vi "CheckUserPass.vi"(6 "password":string, 7 "user":string, 8 "error in":errorcluster, 9 "PasswordRecieved":string, 10 "UserRecieved":string, 11 "connection ID in":refnum<k5>) -> (0 "error out":errorcluster, 3 "connection ID out":refnum<k5>, 5 "result":bool)   [LabVIEW 2010]
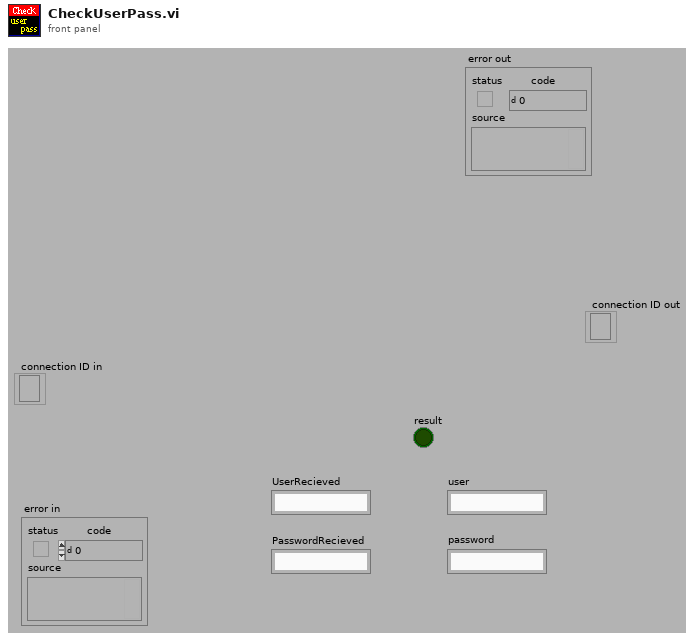
[diagram p1: front panel]
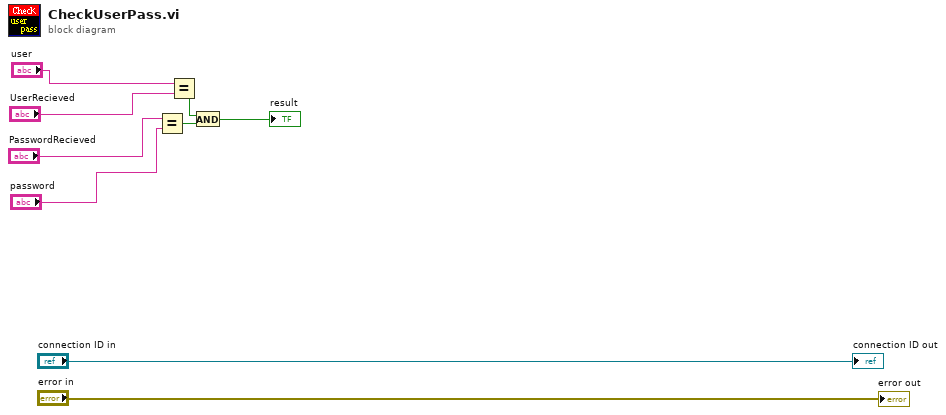
[diagram p0: block diagram]
diagram:
  n1 = Equal?(x="PasswordRecieved", y="password") -> (x = y?=w4:bool)
  n2 = Equal?(x="user", y="UserRecieved") -> (x = y?=w5:bool)
  n3 = And(x=w5, y=w4) -> (x .and. y?=→"result":bool)
  "connection ID out" <- "connection ID in"
  "error out" <- "error in"
